vi "MakeScreenshot(SubVI).vi"(8 "Error In":errorcluster, 10 "String in":refnum<vi>, 11 "VI in":refnum<vi>) -> (0 "Error Out":errorcluster)   [LabVIEW 2018]
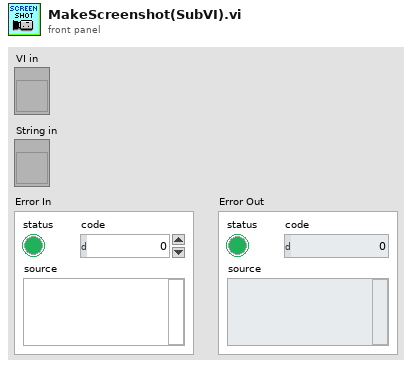
[diagram p1: front panel]
types:
  T1 = typedef "imagedata.ctl" = cluster{"image type":i32, "image depth":i32, "image":u8[], "mask":u8[], "colors":u32[], "Rectangle":cluster{"left":i16, "top":i16, "right":i16, "bottom":i16}}
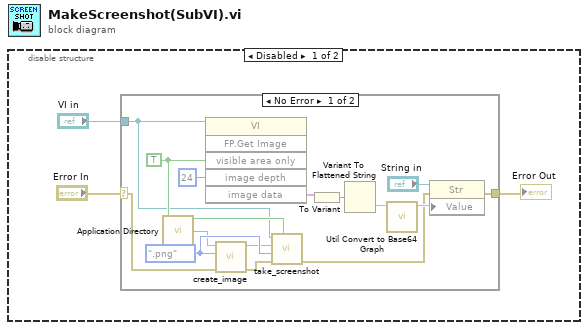
[diagram p0: block diagram]
diagram:
  n1 = disable-structure shown="Disabled" {
    frame Disabled {
      n2 = case shown="No Error" "Error In" {
        selector: "Error In" -> [w5 w19]
        tunnel: [w6 w19] -> w2
        tunnel: "VI in" -> [w4 _]
        frame No Error {
          w14 = TRUE ("Visible Area Only")
          w12 = enum32{".png", ".jpg", ".bmp"}.".png" ("IMG_FORMAT")
          n3 = call <vilib>:"Application Directory.vi"() -> ("Application Directory"=w10:path)
          n4 = invoke class="VI" method="FP.Get Image"(reference=w4, "visible area only"=w14, "image depth"=24 ("Image Depth")) -> ("image data"=w16:T1)  [unwired: 3 in, 5 out]
          n5 = call "create_image.vi"("error in"=w5, "Enum in"=w12, "base path"=w10) -> ("error out"=w8:errorcluster, "path"=w11:path)  [unwired: 7 in]
          n6 = call "take_screenshot.vi"("Visible area only? (f)"=w14, "error in (no error)"=w8, "IMG_FORMAT"=w12, "Image path"=w11, "VI in"=w4) -> ("error out"=w7:errorcluster)  [unwired: 2 in, 1 out]
          n7 = To Variant(anything=w16) -> (Variant=w15:variant)
          n8 = Variant To Flattened String(Variant=w15) -> (data string=w17:string)  [unwired: 1 out]
          n9 = call "Util Convert to Base64 Graph.vi"("String"=w17) -> ("Base64 String"=w18:string)  [unwired: 10 in]
          n10 = property on="Property Node" class="Str"(reference="String in", error in=w7, "Value"=w18) -> (error out=w6:errorcluster)  [unwired: 1 out]
        }
        frame Error {
        }
      }
      "Error Out" <- w2
    }
    frame Enabled {
    }
  }
